vi "Exercise 3-9.vi"() -> ()   [LabVIEW 2014]
panel:
  in  "Max Wind Speed":dbl
  in  "Current Wind Speed":dbl
  in  "Current Temp":dbl
  out "Warning?":bool
  out "Warning Text":string
  in  "Min Temp":dbl
  in  "Max Temp":dbl
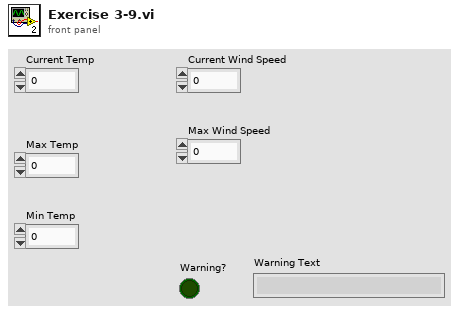
[diagram p1: front panel]
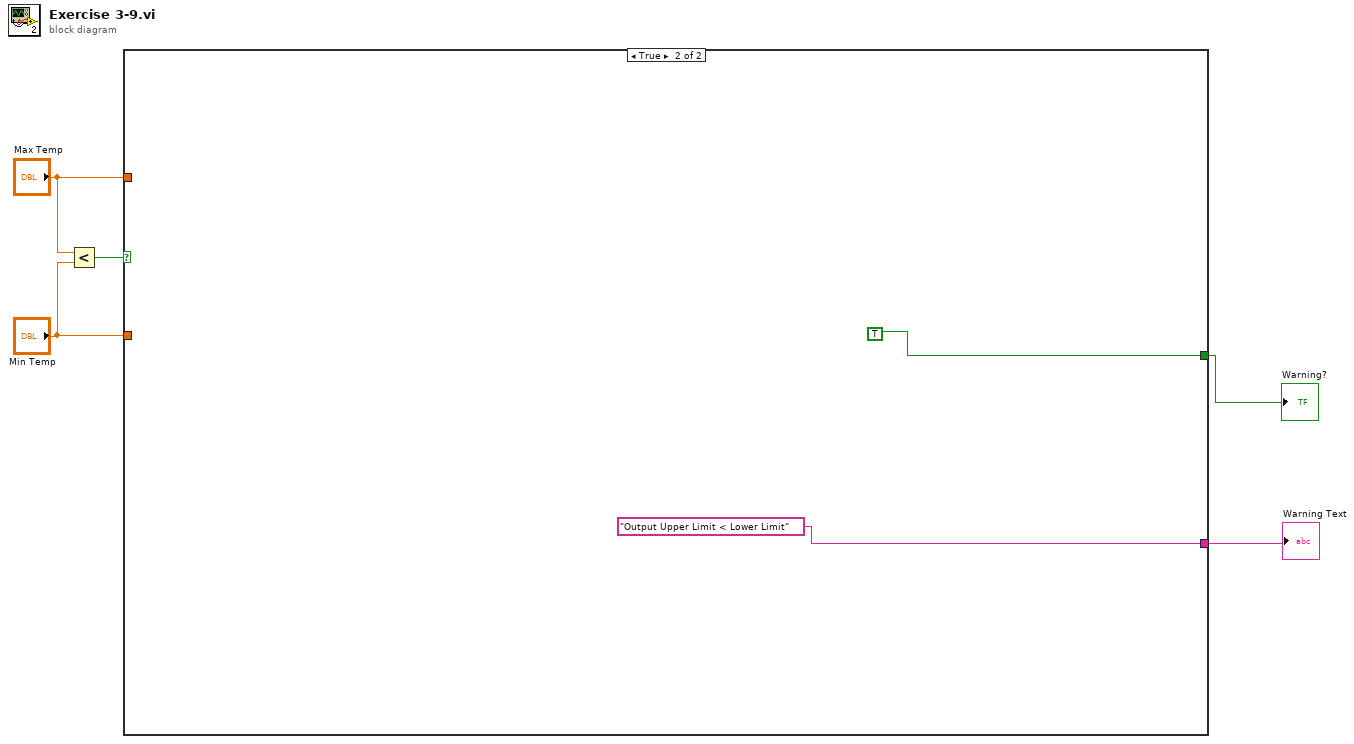
[diagram p0: block diagram]
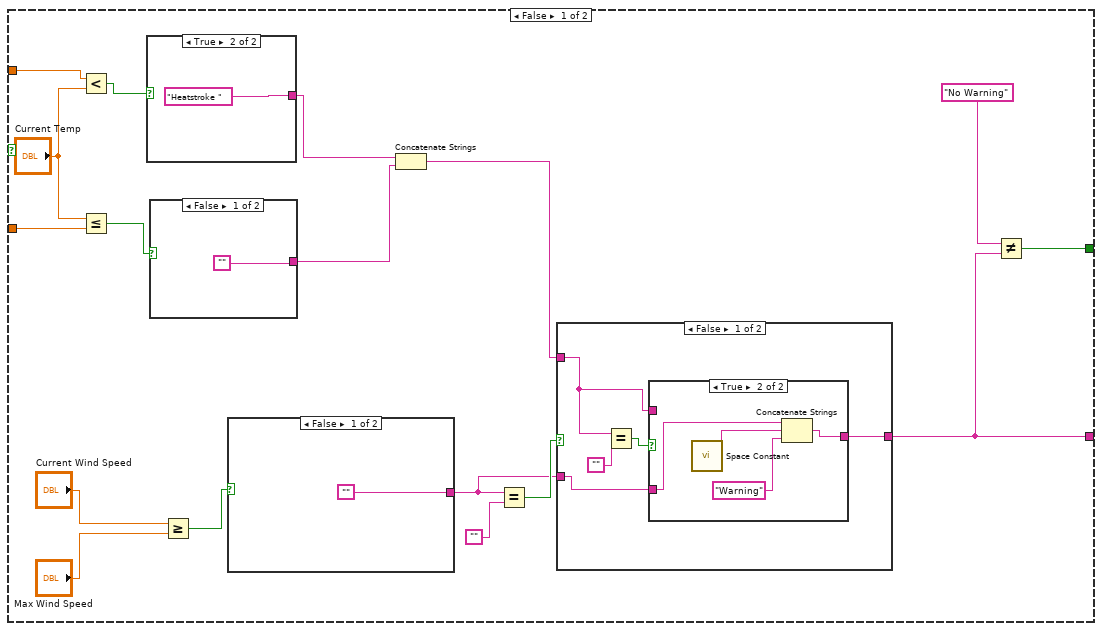
[diagram p2: hidden frame]
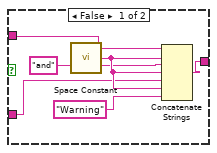
[diagram p3: hidden frame]
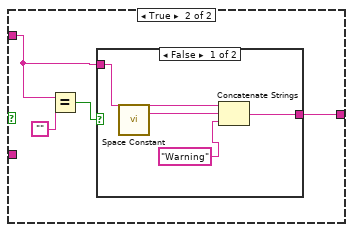
[diagram p4: hidden frame]
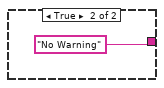
[diagram p5: hidden frame]
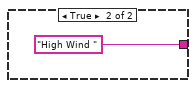
[diagram p6: hidden frame]
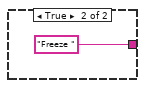
[diagram p7: hidden frame]
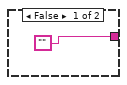
[diagram p8: hidden frame]
diagram:
  n1 = Less?(x="Max Temp", y="Min Temp") -> (x < y?=w5:bool)
  n2 = case shown="True" w5 {
    tunnel: "Max Temp" -> [w8 _]
    tunnel: "Min Temp" -> [w9 _]
    tunnel: [w7 TRUE] -> w1
    tunnel: [w6 "Output Upper Limit < Lower Limit"] -> w2
    frame False {
      n3 = Less?(x=w8, y="Current Temp") -> (x < y?=w21:bool)
      n4 = Less Or Equal?(x="Current Temp", y=w9) -> (x <= y?=w20:bool)
      n5 = case shown="True" w21 {
        tunnel: ["" "Heatstroke "] -> w19
        frame False {
        }
        frame True {
        }
      }
      n6 = case shown="False" w20 {
        tunnel: ["" "Freeze "] -> w18
        frame False {
        }
        frame True {
        }
      }
      n7 = Greater Or Equal?(x="Current Wind Speed", y="Max Wind Speed") -> (x >= y?=w15:bool)
      n8 = case shown="False" w15 {
        tunnel: ["" "High Wind "] -> w12
        frame False {
        }
        frame True {
        }
      }
      n9 = Concatenate Strings(w19, w18) -> (w11:string)
      n10 = Equal?(x=w12, y="") -> (x = y?=w13:bool)
      n11 = case shown="False" w13 {
        tunnel: w12 -> [w24 _]
        tunnel: w11 -> [w26 w39]
        tunnel: [w23 w38] -> w6
        frame False {
          n12 = Equal?(x=w26, y="") -> (x = y?=w25:bool)
          n13 = case shown="True" w25 {
            tunnel: w26 -> [w30 _]
            tunnel: w24 -> [w28 w37]
            tunnel: [w29 w34] -> w23
            frame False {
              n14 = call <vilib>:"Space Constant.vi"() -> ("String"=w32:string)
              n15 = Concatenate Strings(w30, w32, "and", w32, w28, w32, "Warning") -> (w29:string)
            }
            frame True {
              n16 = call <vilib>:"Space Constant.vi"() -> ("String"=w36:string)
              n17 = Concatenate Strings(w37, w36, "Warning") -> (w34:string)
            }
          }
        }
        frame True {
          n18 = Equal?(x=w39, y="") -> (x = y?=w40:bool)
          n19 = case shown="False" w40 {
            tunnel: w39 -> [w43 _]
            tunnel: [w42 "No Warning"] -> w38
            frame False {
              n20 = call <vilib>:"Space Constant.vi"() -> ("String"=w44:string)
              n21 = Concatenate Strings(w43, w44, "Warning") -> (w42:string)
            }
            frame True {
            }
          }
        }
      }
      n22 = Not Equal?(x="No Warning", y=w6) -> (x != y?=w7:bool)
    }
    frame True {
    }
  }
  "Warning Text" <- w2
  "Warning?" <- w1
